vi "Standardize Angle in Radians.vi"(3 "angle in (rad)":dbl, 4 "range (-pi to pi)":T1=enum."-pi to pi") -> (5 "angle out (rad)":dbl)   [LabVIEW 2017, in "NI_Robotics Utilities.lvlib"]
doc: "Wraps an angle in radians to be within a specific range.\n\nThis VI is deprecated. Use <vi.lib>\\Analysis\\coordinate.llb\\Wrap Angle.vi instead."
uses:
  <vilib>/robotics/Utilities/NI_Robotics Utilities.lvlib
  <vilib>/robotics/Utilities/Angle Range_Radians.ctl
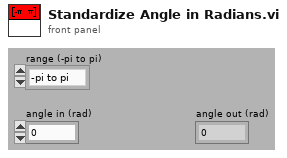
[diagram p1: front panel]
types:
  T1 = typedef "NI_Robotics Utilities.lvlib/Angle Range_Radians.ctl" = enum16{"none", "-pi to pi", "0 to 2*pi"}
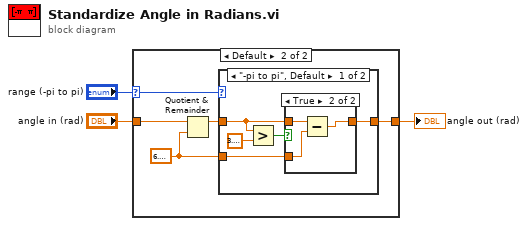
[diagram p0: block diagram]
diagram:
  n1 = case shown="Default" "range (-pi to pi)" {
    selector: "range (-pi to pi)" -> [_ w5]
    tunnel: "angle in (rad)" -> [w4 w8]
    tunnel: [w4 w7] -> w2
    frame "none" {
    }
    frame Default {
      w6 = 6.283185307179586
      n2 = Quotient & Remainder(x=w8, y=w6) -> (x-y*floor(x/y)=w9:dbl)  [unwired: 1 out]
      n3 = case shown="\"-pi to pi\", Default" w5 {
        tunnel: w9 -> [w14 w19]
        tunnel: [w11 w19] -> w7
        tunnel: w6 -> [w10 _]
        frame "-pi to pi", Default {
          n4 = Greater?(x=w14, y=3.141592653589793) -> (0:w12:bool)
          n5 = case shown="True" w12 {
            tunnel: w14 -> [w15 w18]
            tunnel: [w15 w17] -> w11
            tunnel: w10 -> [_ w16]
            frame False {
            }
            frame True {
              n6 = Subtract(x=w18, y=w16) -> (x-y=w17:dbl)
            }
          }
        }
        frame "0 to 2*pi" {
        }
      }
    }
  }
  "angle out (rad)" <- w2
